vi "Get Control Value By Name.vi"(8 "Error In":errorcluster, 10 "key":string, 11 "Map":map{string, refnum<vi>}(c390)) -> (0 "Error Out":errorcluster, 2 "Value":variant, 3 "UIRefsMap":map{string, refnum<vi>}(c390))   [LabVIEW 2019, in "Utilities.lvlib"]
uses:
  Utilities.lvlib
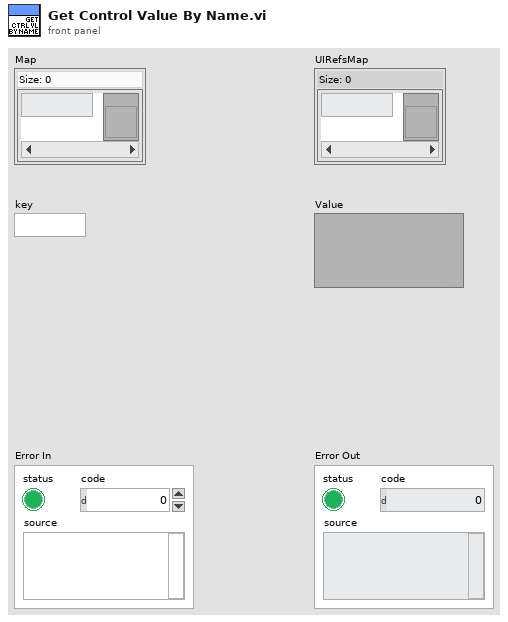
[diagram p1: front panel]
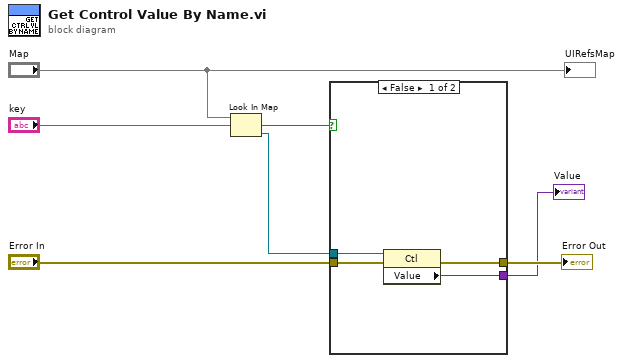
[diagram p0: block diagram]
diagram:
  n1 = Look In Map(map="Map", key="key") -> (key not found?=w2:bool, value=w3:refnum<vi>)  [unwired: 1 in]
  n2 = case shown="False" w2 {
    tunnel: "Error In" -> [w11 w12]
    tunnel: [w10 w12] -> w4
    tunnel: w3 -> [w9 _]
    tunnel: [w8 _] -> w1
    frame False {
      n3 = property class="Ctl"(reference=w9, error in=w11) -> (error out=w10:errorcluster, "Value"=w8:variant)  [unwired: 1 out]
    }
    frame True {
    }
  }
  "Error Out" <- w4
  "Value" <- w1
  "UIRefsMap" <- "Map"
